vi "Handle Error.vi"(8 "error in (no error)":errorcluster, 11 "IMediator In":refnum<class "IMediator.lvclass">) -> (0 "error out":errorcluster, 2 "stop actor?":bool=TRUE, 3 "IMediator Out":refnum<class "IMediator.lvclass">)   [LabVIEW 2018, in "MVA Framework.lvlib" / "IMediator.lvlib" / "IMediator.lvclass"]
doc: "(<B>Filename</B>: Actor Framework.lvlib:Actor.lvclass:Handle Error.vi)\n\nDefines how the actor handles an error that occurred while processing a message. By default, this method does nothing except stop the actor."
uses:
  IMediator.lvclass
  composed-event-logger/Source/Composed Log/Types/Log Level.ctl
  composed-event-logger/Source/Composed Log/Composed Log.lvlib
  <vilib>/ActorFramework/Actor/Actor.lvclass
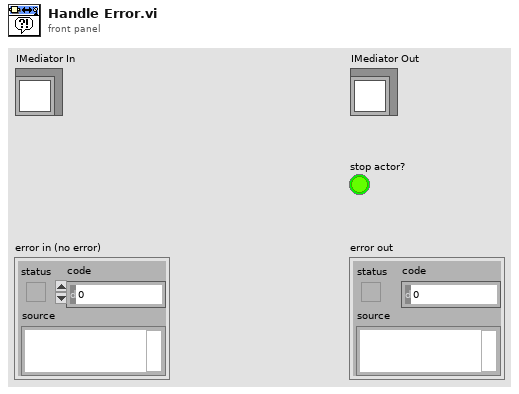
[diagram p1: front panel]
types:
  T1 = typedef "MVA Framework.lvlib/Composed Log.lvlib/Log Level.ctl" = enum16{"Debug", "Info", "Warning", "Error", "Critical"}
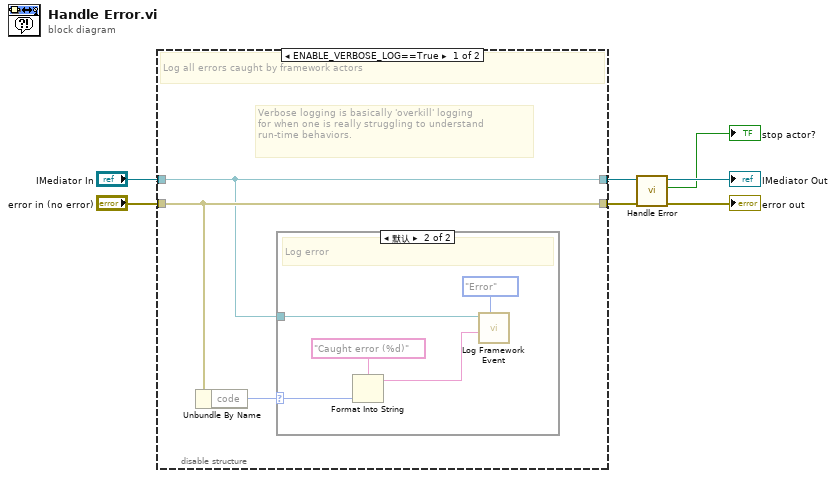
[diagram p0: block diagram]
diagram:
  n1 = disable-structure shown="ENABLE_VERBOSE_LOG==True" {
    disable-tunnel: "IMediator In" -> [w8 w17]
    disable-tunnel: [w8 w17] -> w2
    disable-tunnel: "error in (no error)" -> [w10 w16]
    disable-tunnel: [w10 w16] -> w1
    frame condition #0 {
      # "Verbose logging is basically 'overkill' logging\nfor when one is really struggling to understand\nrun-time behaviors."
      # "Log all errors caught by framework actors"
      n2 = Unbundle By Name(w10) -> ("code"=w9:i32)
      n3 = case shown="默认" w9 {
        selector: w9 -> [_ w14]
        tunnel: w8 -> [_ w13]
        frame 43 {
          # "Normal shutdown -- Do not log"
        }
        frame Default {
          # "Log error"
          n4 = Format Into String(format string="Caught error (%d)", w14) -> (resulting string=w11:string)  [unwired: 2 in, 1 out]
          n5 = call "Log Framework Event.vi"("Event Level (Debug)"=Log_Level."Error", "Data To Log"=w11, "IMediator In"=w13) -> ()  [unwired: 8 in, 1 out]
        }
      }
    }
    frame condition #1 (active) {
      # "Remove all logging from this method at compile time"
    }
  }
  n6 = call-parent "Handle Error.vi"("error in (no error)"=w1, "Actor in"=w2) -> ("error out"=→"error out":errorcluster, "stop actor?"=→"stop actor?":bool, "Actor out"=→"IMediator Out":refnum<class "IMediator.lvclass">)  [unwired: 7 in]
